vi "Configure Multi Batch Text.vi"(0 "VISA resource name":refnum<visa-resource-name>, 1 "Batch Group Number  [/BT] (1)":i32=1 min=1 max=12, 2 "Field Number (1)":i32=1 min=1 max=24, 3 "Title":string, 4 "Text":string, 5 "error in (no error)":errorcluster) -> (14 "VISA resource name out":refnum<visa-resource-name>, 15 "Batch Group Number":i32, 16 "Field Number":i32, 19 "error out":errorcluster)   [LabVIEW 2020, in "Yokogawa GX Series.lvlib"]
doc: "Sets the multi batch text.\n\nCommand: SMltTextField"
uses:
  <instrlib>/Yokogawa GX Series/Yokogawa GX Series.lvlib
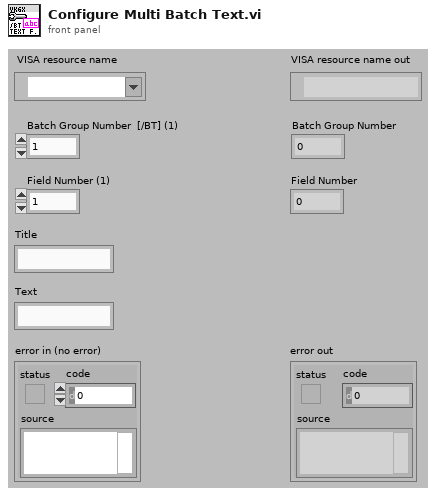
[diagram p1: front panel]
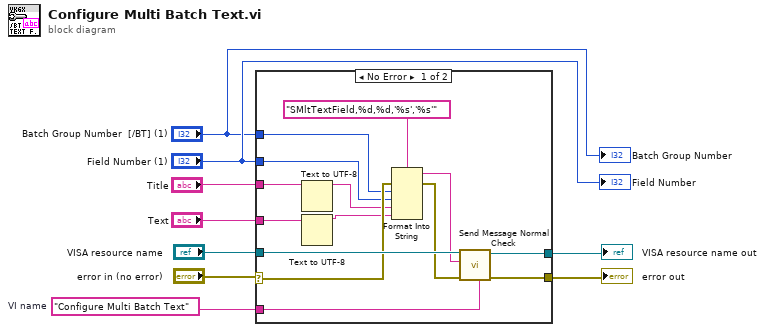
[diagram p0: block diagram]
diagram:
  w8 = "Configure Multi Batch Text"  # VI name
  n1 = case shown="No Error" "error in (no error)" {
    selector: "error in (no error)" -> [w16 w24]
    tunnel: "VISA resource name" -> [w23 w25]
    tunnel: w8 -> [w22 _]
    tunnel: [w21 w25] -> w7
    tunnel: [w20 w24] -> w6
    tunnel: "Field Number (1)" -> [w11 _]
    tunnel: "Title" -> [w14 _]
    tunnel: "Text" -> [w15 _]
    tunnel: "Batch Group Number  [/BT] (1)" -> [w10 _]
    frame No Error {
      n2 = Text to UTF-8(11:w14) -> (3:w12:string)  [unwired: 2 in, 1 out]
      n3 = Text to UTF-8(11:w15) -> (3:w13:string)  [unwired: 2 in, 1 out]
      n4 = Format Into String(format string="SMltTextField,%d,%d,'%s','%s'", error in=w16, w10, w11, w12, w13) -> (resulting string=w18:string, error out=w17:errorcluster)  [unwired: 1 in]
      n5 = call <instrlib>:"Send Message Normal Check.vi"("Source (\"\")"=w22, "error in (no error)"=w17, "Send Message (\"\")"=w18, "VISA resource name"=w23) -> ("error out"=w20:errorcluster, "VISA resource name out"=w21:refnum<visa-resource-name>)  [unwired: 2 in, 4 out]
    }
    frame Error {
    }
  }
  "error out" <- w6
  "VISA resource name out" <- w7
  "Field Number" <- "Field Number (1)"
  "Batch Group Number" <- "Batch Group Number  [/BT] (1)"
